vi "getDOChannel.vi"(8 "error in (no error)":errorcluster, 11 "DoDeviceData.lvclass in":refnum<class "DoDeviceData.lvclass">) -> (0 "error out":errorcluster, 2 "DigitalOutput":refnum<class "DigitalOutput.lvclass">, 3 "DoDeviceData.lvclass out":refnum<class "DoDeviceData.lvclass">)   [LabVIEW 2009, in "DataMappers.lvlib" / "DoDeviceData.lvclass"]
uses:
  DoDeviceData.lvclass
  Hal/Channels/Digital/DigitalOutput.lvclass
  DoDeviceData.lvclass/DoDeviceData.ctl
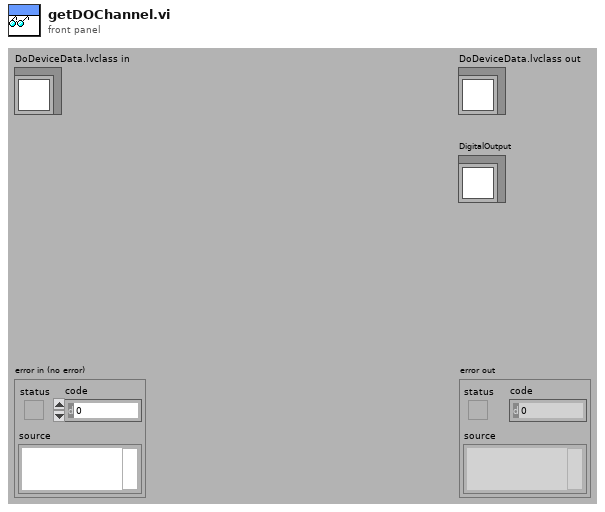
[diagram p1: front panel]
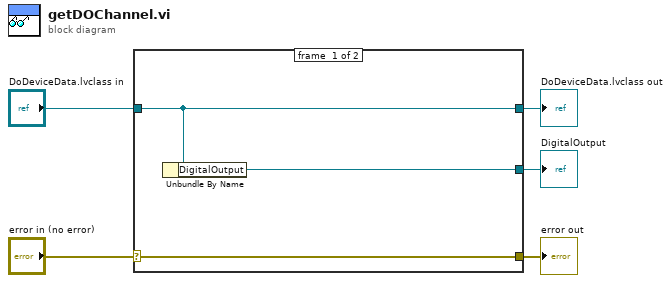
[diagram p0: block diagram]
diagram:
  n1 = case shown="No Error" "error in (no error)" {
    selector: "error in (no error)" -> [w8 w9]
    tunnel: [w8 w9] -> w4
    tunnel: [w7 w10] -> w2
    tunnel: "DoDeviceData.lvclass in" -> [w7 w10]
    tunnel: [w6 _] -> w1
    frame #0 {
      n2 = Unbundle By Name(w7) -> ("DigitalOutput"=w6:refnum<class "DigitalOutput.lvclass">)
    }
    frame #1 {
    }
  }
  "error out" <- w4
  "DoDeviceData.lvclass out" <- w2
  "DigitalOutput" <- w1
